vi "Get camera from cluster.vi"(8 "Error In":errorcluster, 9 "Camera":u8(ring) items=["Red", "Green", "Blue", "UV"], 11 "Camera cluster":T1) -> (0 "Error Out":errorcluster, 3 "Camera reference out":refnum<k24>)   [LabVIEW 2017]
uses:
  C:/Program Files/National Instruments/LabVIEW 2017/instr.lib/IDS/ueye.NET/uEyeDotNet.dll
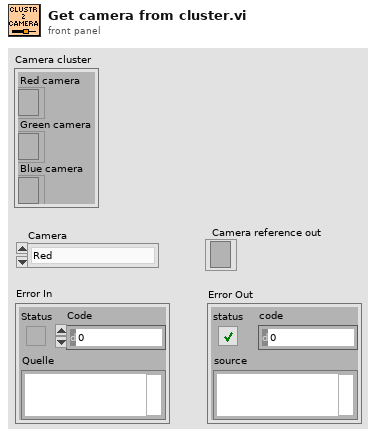
[diagram p1: front panel]
types:
  T1 = cluster{"Red camera":refnum<k24>, "Green camera":refnum<k24>, "Blue camera":refnum<k24>}
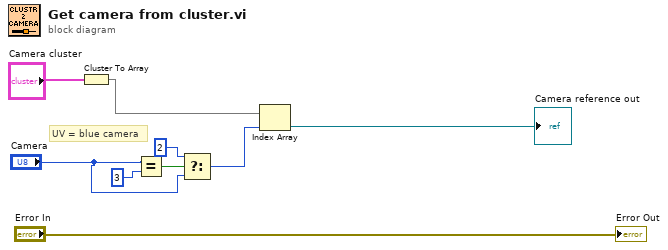
[diagram p0: block diagram]
diagram:
  # "UV = blue camera"
  n1 = Cluster To Array(cluster="Camera cluster") -> (array=w8:refnum<k24>[])
  n2 = Equal?(x="Camera", y=u8 3) -> (x = y?=w4:bool)
  n3 = Select(t=u8 2, s=w4, f="Camera") -> (s? t:f=w2:u8)
  n4 = Index Array(array=w8, index=w2) -> (element=→"Camera reference out":refnum<k24>)
  "Error Out" <- "Error In"
